vi "Set Heater.vi"(6 "Channel":i32, 8 "error in (no error)":errorcluster, 10 "Current (A)":dbl, 11 "Instrument.Cryostat in":refnum<class "Instrument.Cryostat.lvclass">) -> (0 "error out":errorcluster, 3 "Instrument.Cryostat out":refnum<class "Instrument.Cryostat.lvclass">)   [LabVIEW 2019, in "Instrument.Cryostat.lvclass"]
uses:
  Instrument.Cryostat.lvclass
  Typedefs/Set Heater--cluster.ctl
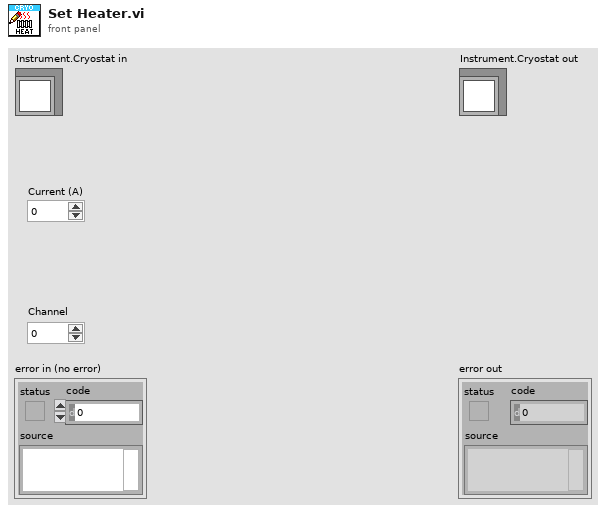
[diagram p1: front panel]
types:
  T1 = typedef "Instrument.Cryostat.lvclass/Set Heater--cluster.ctl" = cluster{"Channel":i32, "Current (A)":dbl}
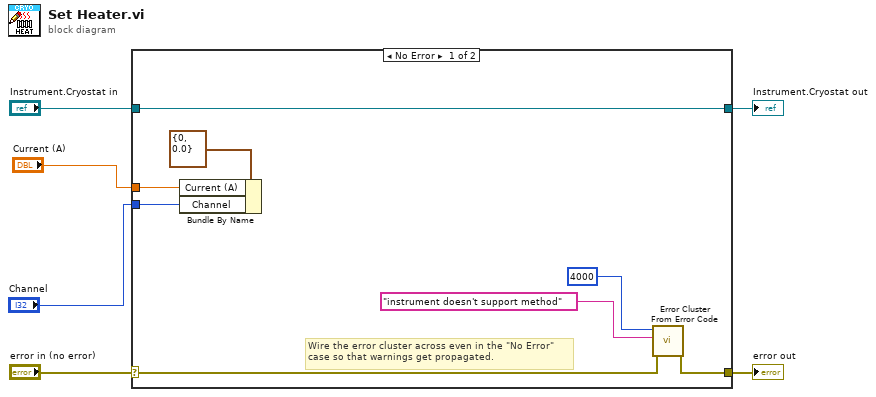
[diagram p0: block diagram]
diagram:
  n1 = case shown="No Error" "error in (no error)" {
    selector: "error in (no error)" -> [w11 w16]
    tunnel: [w10 w16] -> w5
    tunnel: [w14 w15] -> w3
    tunnel: "Instrument.Cryostat in" -> [w14 w15]
    tunnel: "Current (A)" -> [w9 _]
    tunnel: "Channel" -> [w8 _]
    frame No Error {
      # "Wire the error cluster across even in the \"No Error\"\ncase so that warnings get propagated."
      n2 = Bundle By Name(cluster=T1 {"Channel"=0, "Current (A)"=0.0} ("Set Temperature"), "Current (A)"=w9, "Channel"=w8) -> ()  [unwired: 1 out]
      n3 = call <vilib>:"Error Cluster From Error Code.vi"("error in (no error)"=w11, "error message (\"\")"="instrument doesn't support method" ("error message (\"\")"), "error code (0)"=4000) -> ("error out"=w10:errorcluster)  [unwired: 6 in]
    }
    frame Error {
    }
  }
  "error out" <- w5
  "Instrument.Cryostat out" <- w3
